vi "Update Channel Enum.vi"(8 "error in (no error)":errorcluster, 11 "Path to Common Folder":path=path "D:/dev/CIF-LVCore/src/CIFTemplatePlugin/Common") -> (0 "error out":errorcluster)   [LabVIEW 2021, in "CIFChannelMng.lvclass"]
uses:
  CIFChannelMng.lvclass
  CIFUtilities/Scripting/Update Enum/typdef/ControlTypes.ctl
  <userlib>/_OpenG.lib/lvdata/lvdata.llb/openg_variant.lvlib
  CIFUtilities/Scripting/Update Enum/Update Enum.lvlib
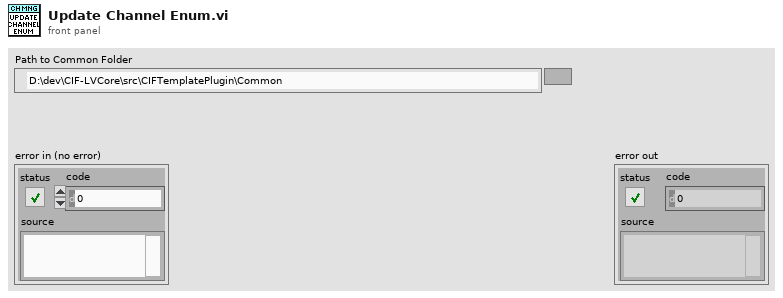
[diagram p1: front panel]
types:
  T1 = typedef "ChannelRegistrar.lvlib/Channel Definition.ctl" = cluster{"Name":string, "Direction":T2, "Type":T3, "Custom Config Data":u8[]}
  T2 = typedef "CIFChannels.lvclass/Direction.ctl" = enum16{"Publisher", "Subscriber"}
  T3 = typedef "ChannelRegistrar.lvlib/Registered Channel Types.ctl" = u16
  T4 = typedef "Update Enum.lvlib/ControlTypes.ctl" = enum32{"not a control VI", "control", "typedef", "strict typedef"}
  T5 = enum32{"invalid VI type", "Standard VI", "Control VI", "Global VI", "Polymorphic VI"}
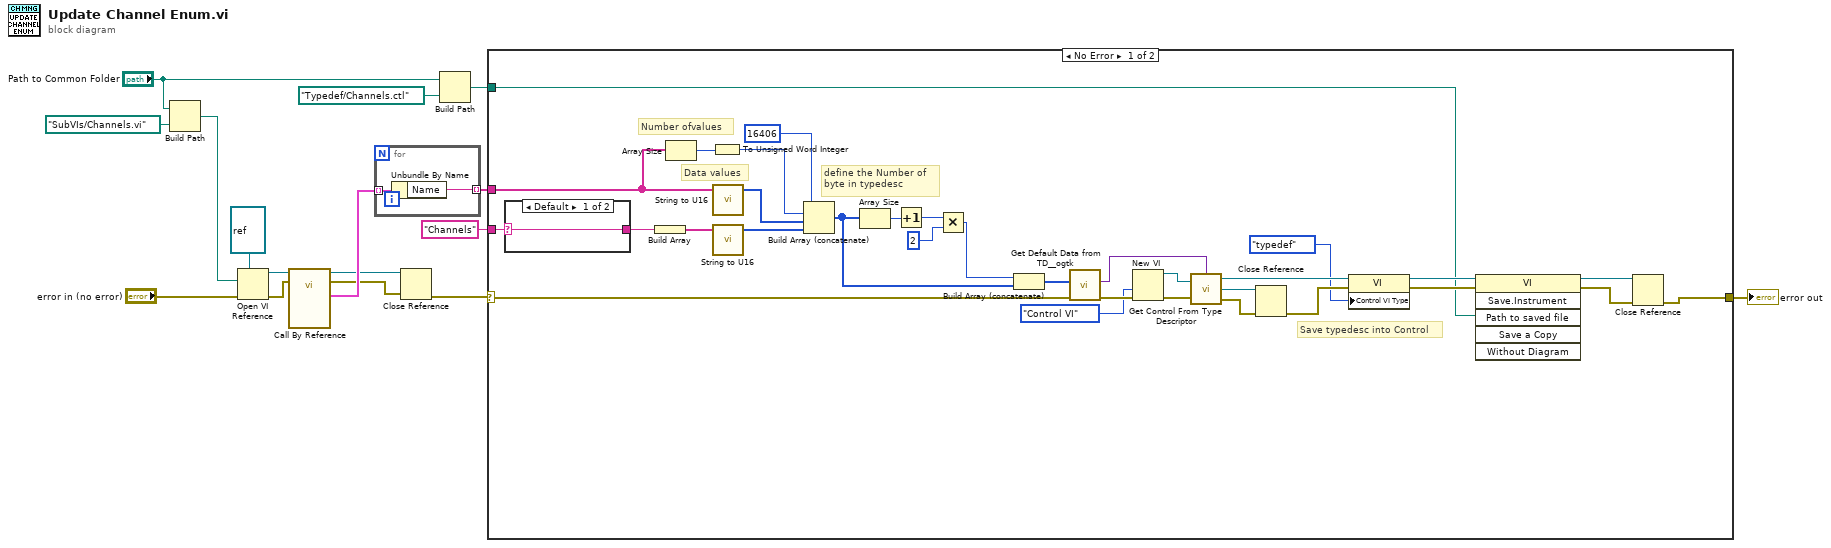
[diagram p0: block diagram]
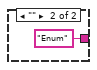
[diagram p2: hidden frame]
diagram:
  n1 = Build Path(base path="Path to Common Folder", name or relative path=path "SubVIs/Channels.vi") -> (appended path=w5:path)
  n2 = Open VI Reference(type specifier VI Refnum (for type only)=refnum<vi> refnum, vi path=w5, error in (no error)="error in (no error)") -> (vi reference=w12:refnum<vi>, error out=w11:errorcluster)  [unwired: 3 in]
  n3 = call-by-ref "?"(reference=w12, error in=w11) -> (reference out=w9:refnum<vi>, error out=w8:errorcluster, "Channels to Create"=w10:T1[])  [unwired: 11 in]
  n4 = for {
    tunnel: w10 -> [w18] mode=indexing
    tunnel: [w17] -> w14 mode=indexing
    n5 = Unbundle By Name(w18) -> ("Name"=w17:string)
  }
  n6 = Close Reference(reference=w9, error in (no error)=w8) -> (error out=w7:errorcluster)
  n7 = Build Path(base path="Path to Common Folder", name or relative path=path "Typedef/Channels.ctl") -> (appended path=w2:path)
  n8 = case shown="No Error" w7 {
    selector: w7 -> [w39 w53]
    tunnel: w14 -> [w38 _]
    tunnel: "Channels" ("Enum Name (Enum)") -> [w50 _]
    tunnel: [w26 w53] -> w16
    tunnel: w2 -> [w24 _]
    frame No Error {
      # "Save typedesc into Control"
      # "Data values"
      # "Number ofvalues"
      # "define the Number of\nbyte in typedesc"
      n9 = case shown="Default" w50 {
        selector: w50 -> [w51 _]
        tunnel: [w51 "Enum"] -> w41
        frame Default {
        }
        frame "" {
        }
      }
      n10 = Build Array(w41) -> (w36:string[])
      n11 = Array Size(array=w38) -> (size(s)=w43:i32)
      n12 = To Unsigned Word Integer(number=w43) -> (unsigned 16bit integer=w42:u16)
      n13 = call "String to U16.vi"("Array of Strings"=w38) -> ("Array of U16"=w37:u16[])  [unwired: 4 in]
      n14 = call "String to U16.vi"("Array of Strings"=w36) -> ("Array of U16"=w35:u16[])  [unwired: 4 in]
      n15 = Build Array (concatenate)(u16 16406, w42, w37, w35) -> (w45:u16[])
      n16 = Array Size(array=w45) -> (size(s)=w49:i32)
      n17 = Increment(x=w49) -> (x+1=w48:i32)
      n18 = Multiply(x=w48, y=2) -> (x*y=w46:i32)
      n19 = Build Array (concatenate)(w46, w45) -> (w40:i32[])
      n20 = call <userlib>:"Get Default Data from TD__ogtk.vi"("error in (no error)"=w39, "Type Descriptor"=w40) -> ("error out"=w27:errorcluster, "Default VData"=w22:variant)  [unwired: 8 in]
      n21 = New VI(8:w27, 9:T5."Control VI" ("vi type (standard vi)")) -> (0:w34:errorcluster, 3:w23:refnum<vi>)  [unwired: 5 in]
      n22 = call "Get Control From Type Descriptor.vi"("VI Refnum"=w23, "error in (no error)"=w34, "data type"=w22) -> ("VI Refnum"=w20:refnum<vi>, "New Control Ref"=w32:refnum<vi>, "error out"=w31:errorcluster)
      n23 = Close Reference(reference=w32, error in (no error)=w31) -> (error out=w30:errorcluster)
      n24 = property class="VI"(reference=w20, error in=w30, "Control VI Type"=ControlTypes."typedef" ("Control VI Type (control)")) -> (reference out=w28:refnum<vi>, error out=w29:errorcluster)
      n25 = invoke class="VI" method="Save.Instrument"(reference=w28, error in=w29, "Path to saved file"=w24) -> (reference out=w33:refnum<vi>, error out=w25:errorcluster)  [unwired: 3 in, 4 out]
      n26 = Close Reference(reference=w33, error in (no error)=w25) -> (error out=w26:errorcluster)
    }
    frame Error {
    }
  }
  "error out" <- w16
